vi "FRA_UDP_send_ACK.vi"() -> (3 "Datagram to send":string)   [LabVIEW 2013]
doc: "Sends GMT time and ACK"
panel:
  out "output array":u8[](array[numeric]) format="%x"
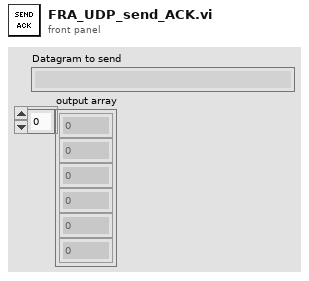
[diagram p1: front panel]
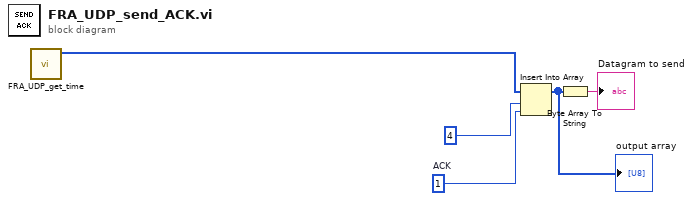
[diagram p0: block diagram]
diagram:
  w2 = u8 1  # ACK
  n1 = call "FRA_UDP_get_time.vi"() -> ("array"=w3:u8[])  [unwired: 11 in]
  n2 = Insert Into Array(array=w3, index=4, new element=w2) -> (w1:u8[])
  "output array" <- w1
  n3 = Byte Array To String(unsigned byte array=w1) -> (string=→"Datagram to send":string)
